vi "Form GSA Sentence.vi"(8 "error in (no error)":errorcluster, 11 "GSA data":T1={"selection of fix"={"included?"=TRUE, "selection of 2D or 3D fix"=0}, "type of fix"={"included?"=TRUE, "mode"=0}, "satellite PRN numbers"={"included?"=[TRUE, TRUE, TRUE, TRUE, TRUE, TRUE, TRUE, TRUE, TRUE, TRUE, TRUE, TRUE], "PRN numbers"=[]}, "dilution of precision"={"included?"=TRUE, "DOP"=0.0}, "horizontal dilution of precision"={"included?"=TRUE, "horizontal DOP"=0.0}, "vertical dilution of precision"={"included?"=TRUE, "vertical DOP"=0.0}} {"type of fix"."mode" items=["", "No Fix", "2D Fix", "3D Fix"]; "selection of fix"."selection of 2D or 3D fix" items=["Automatic", "Manual"]}) -> (0 "error out":errorcluster, 3 "GSA sentence":string)   [LabVIEW 2011, in "u-blox 5 Series.lvlib"]
doc: "Creates an NMEA sentence using the data you specify for a particular sentence type. You must manually select the polymorphic instance to use."
uses:
  u-blox 5 Series.lvlib
  typedefs/GSA Data.ctl
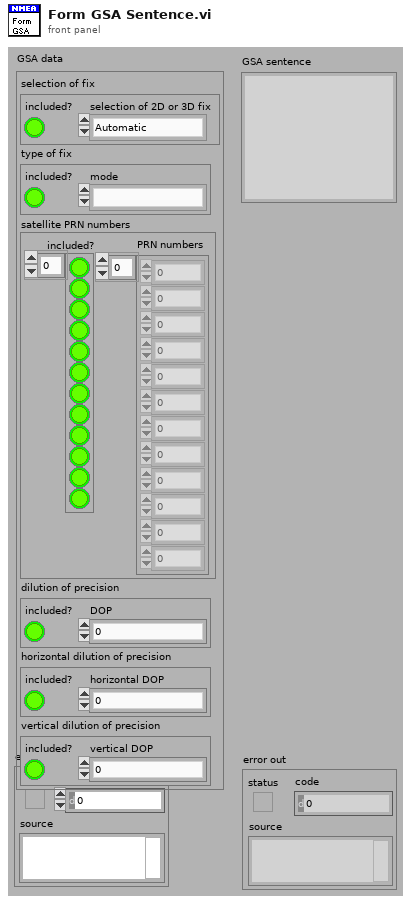
[diagram p1: front panel]
types:
  T1 = typedef "u-blox 5 Series.lvlib/GSA Data.ctl" = cluster{"selection of fix":cluster{"included?":bool, "selection of 2D or 3D fix":u16}, "type of fix":cluster{"included?":bool, "mode":u16}, "satellite PRN numbers":cluster{"included?":bool[], "PRN numbers":i32[]}, "dilution of precision":cluster{"included?":bool, "DOP":dbl}, "horizontal dilution of precision":cluster{"included?":bool, "horizontal DOP":dbl}, "vertical dilution of precision":cluster{"included?":bool, "vertical DOP":dbl}}
  T2 = cluster{"included?":bool, "selection of 2D or 3D fix":u16}
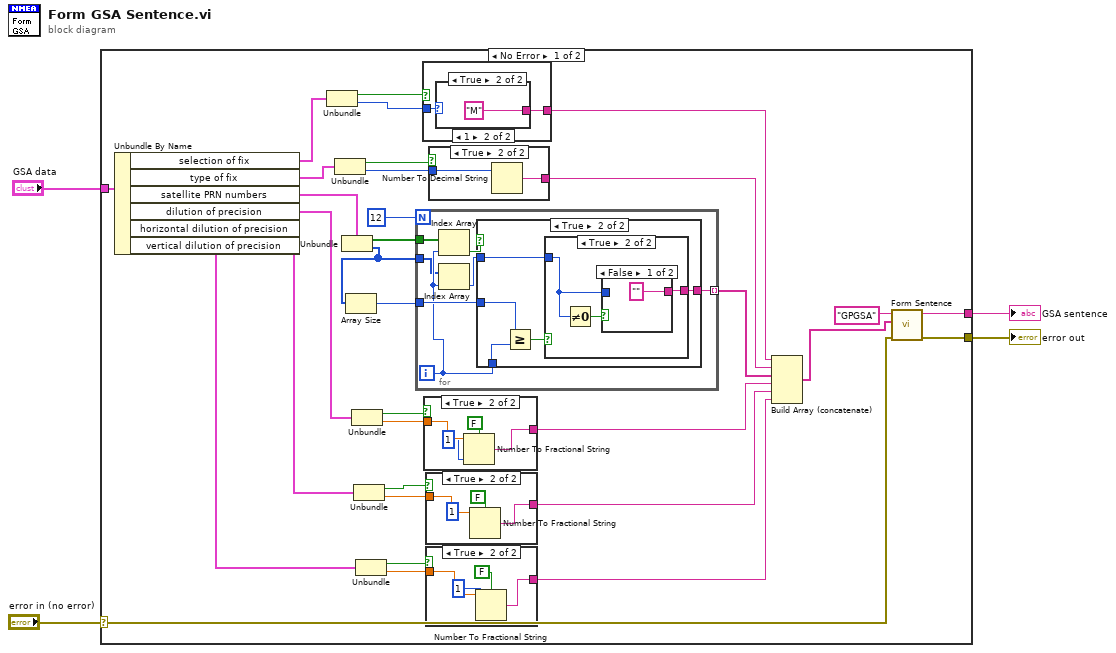
[diagram p0: block diagram]
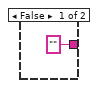
[diagram p2: hidden frame]
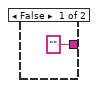
[diagram p3: hidden frame]
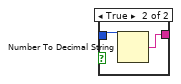
[diagram p4: hidden frame]
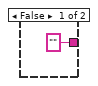
[diagram p5: hidden frame]
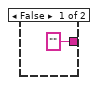
[diagram p6: hidden frame]
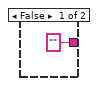
[diagram p7: hidden frame]
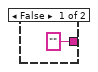
[diagram p8: hidden frame]
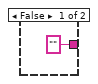
[diagram p9: hidden frame]
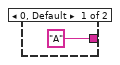
[diagram p10: hidden frame]
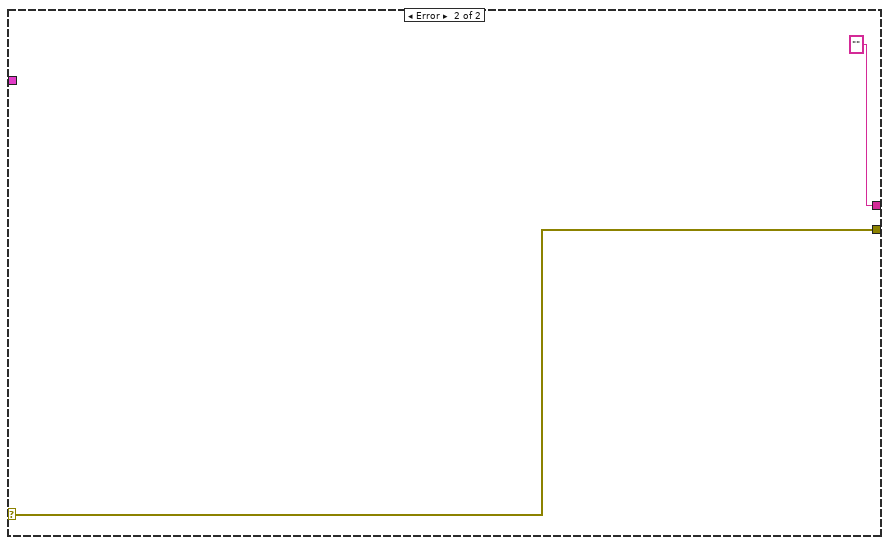
[diagram p11: hidden frame]
diagram:
  n1 = case shown="No Error" "error in (no error)" {
    selector: "error in (no error)" -> [w25 w80]
    tunnel: "GSA data" -> [w36 _]
    tunnel: [w34 w80] -> w1
    tunnel: [w33 "" ("NMEA Sentence")] -> w2
    frame No Error {
      n2 = Unbundle By Name(w36) -> ("selection of fix"=w22:T2, "type of fix"=w21:cluster{"included?":bool, "mode":u16}, "satellite PRN numbers"=w18:cluster{"included?":bool[], "PRN numbers":i32[]}, "dilution of precision"=w16:cluster{"included?":bool, "DOP":dbl}, "horizontal dilution of precision"=w13:cluster{"included?":bool, "horizontal DOP":dbl}, "vertical dilution of precision"=w10:cluster{"included?":bool, "vertical DOP":dbl})
      n3 = Unbundle(w22) -> ("included?"=w23:bool, "selection of 2D or 3D fix"=w24:u16)
      n4 = Unbundle(w21) -> ("included?"=w19:bool, "mode"=w20:u16)
      n5 = Unbundle(w18) -> ("included?"=w5:bool[], "PRN numbers"=w17:i32[])
      n6 = Array Size(array=w17) -> (size(s)=w6:i32)
      n7 = Unbundle(w16) -> ("included?"=w14:bool, "DOP"=w15:dbl)
      n8 = Unbundle(w13) -> ("included?"=w11:bool, "horizontal DOP"=w12:dbl)
      n9 = Unbundle(w10) -> ("included?"=w8:bool, "vertical DOP"=w9:dbl)
      n10 = for {
        N: 12 -> [_]
        tunnel: w17 -> [w39]
        tunnel: [w43] -> w30 mode=indexing
        tunnel: w6 -> [w42]
        tunnel: w5 -> [w40]
        i -> [w41]
        n11 = Index Array(array=w40, index=w41) -> (element=w38:bool)
        n12 = Index Array(array=w39, index=w41) -> (element=w37:i32)
        n13 = case shown="True" w38 {
          tunnel: w37 -> [_ w49]
          tunnel: ["" w48] -> w43
          tunnel: w41 -> [_ w45]
          tunnel: w42 -> [_ w47]
          frame False {
          }
          frame True {
            n14 = Greater Or Equal?(x=w47, y=w45) -> (x >= y?=w46:bool)
            n15 = case shown="True" w46 {
              tunnel: w49 -> [_ w51]
              tunnel: ["" w53] -> w48
              frame False {
              }
              frame True {
                n16 = Not Equal To 0?(x=w51) -> (x != 0?=w52:bool)
                n17 = case shown="False" w52 {
                  tunnel: w51 -> [_ w56]
                  tunnel: ["" w55] -> w53
                  frame False {
                  }
                  frame True {
                    n18 = Number To Decimal String(number=w56) -> (decimal integer string=w55:string)  [unwired: 1 out]
                  }
                }
              }
            }
          }
        }
      }
      n19 = case shown="True" w23 {
        tunnel: ["" w77] -> w32
        tunnel: w24 -> [_ w76]
        frame False {
        }
        frame True {
          n20 = case shown="1" w76 {
            tunnel: ["A" "M"] -> w77
            frame 0, Default {
            }
            frame 1 {
            }
          }
        }
      }
      n21 = case shown="True" w14 {
        tunnel: ["" w71] -> w29
        tunnel: w15 -> [_ w70]
        frame False {
        }
        frame True {
          n22 = Number To Fractional String(use system decimal point (T)=FALSE, number=w70, precision (6)=i16 1) -> (F-format string=w71:string)  [unwired: 1 out]
        }
      }
      n23 = case shown="True" w11 {
        tunnel: ["" w66] -> w28
        tunnel: w12 -> [_ w65]
        frame False {
        }
        frame True {
          n24 = Number To Fractional String(use system decimal point (T)=FALSE, number=w65, precision (6)=i16 1) -> (F-format string=w66:string)  [unwired: 1 out]
        }
      }
      n25 = case shown="True" w8 {
        tunnel: ["" w61] -> w27
        tunnel: w9 -> [_ w60]
        frame False {
        }
        frame True {
          n26 = Number To Fractional String(use system decimal point (T)=FALSE, number=w60, precision (6)=i16 1) -> (F-format string=w61:string)  [unwired: 1 out]
        }
      }
      n27 = case shown="True" w19 {
        tunnel: ["" w74] -> w31
        tunnel: w20 -> [_ w73]
        frame False {
        }
        frame True {
          n28 = Number To Decimal String(number=w73) -> (decimal integer string=w74:string)  [unwired: 1 out]
        }
      }
      n29 = Build Array (concatenate)(w32, w31, w30, w29, w28, w27) -> (w26:string[])
      n30 = call "Form Sentence.vi"("error in (no error)"=w25, "sentence data"=w26, "sentence type"="GPGSA" ("Sentence Type")) -> ("error out"=w34:errorcluster, "sentence"=w33:string)  [unwired: 5 in]
    }
    frame Error {
    }
  }
  "error out" <- w1
  "GSA sentence" <- w2
